vi "refresh stuff.vi"(8 "error in (no error)":errorcluster, 11 "Waveform in":refnum<class "Waveform.lvclass">) -> (0 "error out":errorcluster, 3 "Waveform out":refnum<class "Waveform.lvclass">)   [LabVIEW 2012, in "Waveform.lvclass"]
uses:
  Waveform.lvclass
  Waveform.lvclass/Waveform.ctl
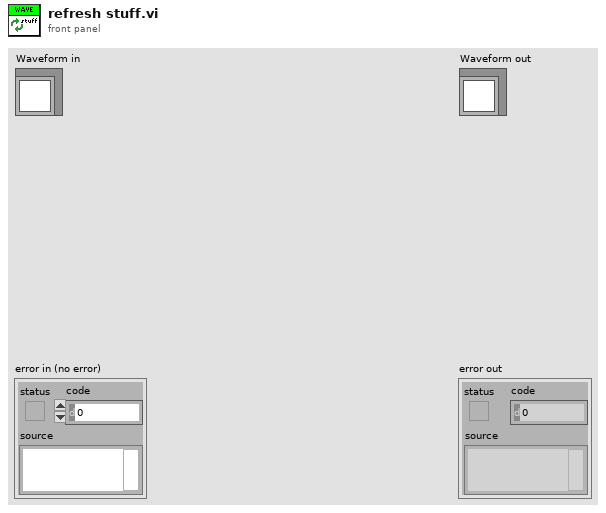
[diagram p1: front panel]
types:
  T1 = typedef "PC_wavelength.ctl" = dbl
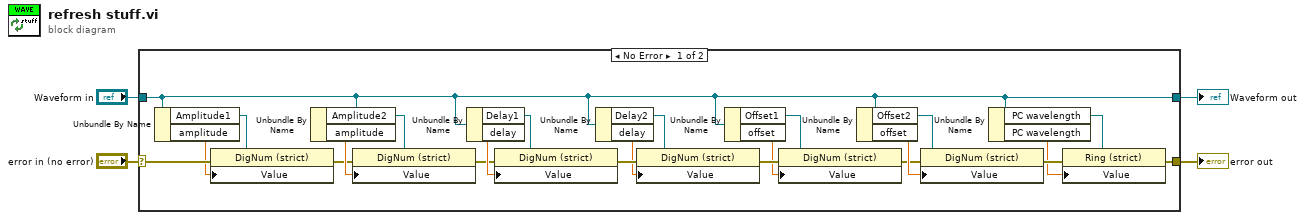
[diagram p0: block diagram]
diagram:
  n1 = case shown="No Error" "error in (no error)" {
    selector: "error in (no error)" -> [w27 w29]
    tunnel: [w5 w29] -> w3
    tunnel: [w9 w28] -> w1
    tunnel: "Waveform in" -> [w9 w28]
    frame No Error {
      n2 = Unbundle By Name(w9) -> ("Amplitude1"=w26:refnum<vi>, "amplitude"=w25:dbl[unit])
      n3 = property class="DigNum (strict)"(reference=w26, error in=w27, "Value"=w25) -> (error out=w20:errorcluster)  [unwired: 1 out]
      n4 = Unbundle By Name(w9) -> ("Amplitude2"=w23:refnum<vi>, "amplitude"=w24:dbl[unit])
      n5 = property class="DigNum (strict)"(reference=w23, error in=w20, "Value"=w24) -> (error out=w19:errorcluster)  [unwired: 1 out]
      n6 = Unbundle By Name(w9) -> ("Delay1"=w21:refnum<vi>, "delay"=w22:dbl[unit])
      n7 = property class="DigNum (strict)"(reference=w21, error in=w19, "Value"=w22) -> (error out=w18:errorcluster)  [unwired: 1 out]
      n8 = Unbundle By Name(w9) -> ("Delay2"=w17:refnum<vi>, "delay"=w16:dbl[unit])
      n9 = property class="DigNum (strict)"(reference=w17, error in=w18, "Value"=w16) -> (error out=w11:errorcluster)  [unwired: 1 out]
      n10 = Unbundle By Name(w9) -> ("Offset1"=w12:refnum<vi>, "offset"=w10:dbl[unit])
      n11 = property class="DigNum (strict)"(reference=w12, error in=w11, "Value"=w10) -> (error out=w13:errorcluster)  [unwired: 1 out]
      n12 = Unbundle By Name(w9) -> ("Offset2"=w14:refnum<vi>, "offset"=w15:dbl[unit])
      n13 = property class="DigNum (strict)"(reference=w14, error in=w13, "Value"=w15) -> (error out=w8:errorcluster)  [unwired: 1 out]
      n14 = Unbundle By Name(w9) -> ("PC wavelength"=w7:refnum<vi>, "PC wavelength"=w6:T1)
      n15 = property class="Ring (strict)"(reference=w7, error in=w8, "Value"=w6) -> (error out=w5:errorcluster)  [unwired: 1 out]
    }
    frame Error {
    }
  }
  "error out" <- w3
  "Waveform out" <- w1
